vi "Write Debug info.vi"(9 "Debug info":string, 11 "CDebugInfo in":refnum<class "CDebugInfo.lvclass">) -> (3 "CDebugInfo out":refnum<class "CDebugInfo.lvclass">)   [LabVIEW 2020, in "DependencyInspection.lvlib" / "CDebugInfo.lvclass"]
uses:
  CDebugInfo.lvclass
  CDebugInfo.lvclass/CDebugInfo.ctl
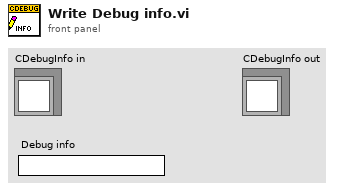
[diagram p1: front panel]
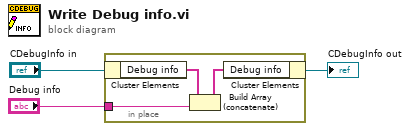
[diagram p0: block diagram]
diagram:
  n1 = in-place {
    in-place-border: "Debug info" -> [w5]
    n2 = in-place-cluster #1("CDebugInfo in") -> ("Debug info"=w6:string[])
    n3 = Build Array (concatenate)(w6, w5) -> (w4:string[])
    n4 = in-place-cluster #1("Debug info"=w4) -> (→"CDebugInfo out":refnum<class "CDebugInfo.lvclass">)
  }
